vi "global_act_eje_aula.vi"() -> ()   [LabVIEW 2017]
panel:
  out "act_aula":bool
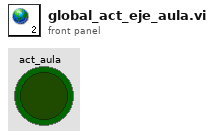
[diagram p1: front panel]
diagram:
